vi "Counter.vi"(5 "ticks":u16) -> (6 "ding":bool)   [LabVIEW 2015]
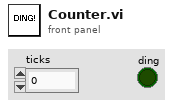
[diagram p1: front panel]
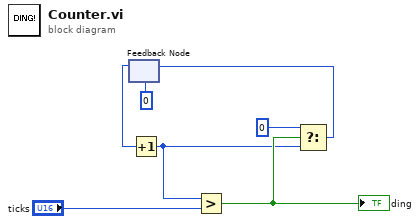
[diagram p0: block diagram]
diagram:
  n1 = feedback #1(u16 0 ("ticks")) -> (w6:u16)
  n2 = Increment(x=w6) -> (x+1=w3:u16)
  n3 = Greater?(x=w3, y="ticks") -> (0:w4:bool)
  "ding" <- w4
  n4 = Select(t=u16 0, s=w4, f=w3) -> (s? t:f=w2:u16)
  n5 = feedback-in #1(w2) -> ()
